vi "CD Init_Prepare Async Data_RT to BC and RT to RT.vi"(8 "error in (no error)":errorcluster, 10 "Card Parameters (in)":T5, 11 "Channels In":T12[](array[typedef]) {"RTs"."Mode Codes"."param item refs" format="%.0x"; "RTs"."Mode Codes"."Timestamp Channel Data Reference" format="%.0x"; "RTs"."subAddresses"."param item refs" format="%.0x"; "RTs"."subAddresses"."Timestamp Channel Data Reference" format="%.0x"; "RTs"."Status Channel Data Reference" format="%.0x"; "RTs"."Command Channels Refs" format="%.0x"; "BC"."Acyclic Frames Trigger Channels Refs" format="%.0x"; "BC"."Command Channels Refs" format="%.0x"; "BC"."messages"."Timestamp Channel Data Reference" format="%.0x"; "BC"."messages"."Status Channel Data Refs" format="%.0x"; "BC"."messages"."param item refs" format="%.0x"; "BC"."messages"."param Block Data Refs"."Data Reference" format="%.0x"}) -> (0 "error out":errorcluster, 1 "param map (RT to BC)":T1, 2 "Raw Values (RT to BC)":T7, 3 "Map (RT to BC)":T9[](array[typedef]) {"Word Data Reference" format="%.0x"})   [LabVIEW 2020, in "Ballard MIL-1553 Engine.lvlib"]
doc: "This VI creates a static association between NI-VS FIFO Channel Index and Physical Channel, Label Index, Parameter Index for Parameter Channel of a Tx Scheduled Label."
uses:
  Ballard MIL-1553 Engine.lvlib
  Shared/Controls and Global/RT Channel.ctl
  Shared/Controls and Global/RT BC.ctl
  <vilib>/NI VeriStand/Custom Device API/Custom Device Item Ref.ctl
  Shared/Controls and Global/RT Message.ctl
  Shared/Controls and Global/RT messageType.ctl
  Shared/Controls and Global/RT CWD1.ctl
  Shared/Controls and Global/RT CWD2.ctl
  <vilib>/NI VeriStand/Custom Device API/Data Reference.ctl
  <vilib>/NI VeriStand/Custom Device API/Block Data Reference.ctl
  System Explorer/SubVIs/Parse Parameters File/param_map_sysdef_type.ctl
  Azdo/emea-ni-vscd_Configurator/source/ConfiguratorConsumer/Ballard_1553/controls/param_type.ctl
  Azdo/emea-ni-vscd_Configurator/source/ConfiguratorConsumer/Ballard_1553/controls/param_signalType_type.ctl
  Azdo/emea-ni-vscd_Configurator/source/ConfiguratorConsumer/Ballard_1553/controls/param_encoding_type.ctl
  Shared/Controls and Global/RT Remote Terminal.ctl
  Shared/Controls and Global/RT Remote Terminal_rtMode.ctl
  Shared/Controls and Global/RT Remote Terminal_RT subAddress.ctl
  Shared/Controls and Global/RT Remote Terminal_RT direction.ctl
  Shared/Controls and Global/RT Remote Terminal_RT Mode Code.ctl
  Controls/RT Async_Map RT2BC.ctl
  Controls/RT Async_Map_Type.ctl
  Controls/RT Async_Raw Values.ctl
  Controls/RT Async_Raw Values to Messages Index_Association.ctl
  Controls/Card Parameters.ctl
  Shared/Controls and Global/Initialization Method.ctl
  Controls/Asynchronous - Parameter map_type.ctl
  Shared/EncodeDecode/_typedefs/parameter_config_type.ctl
  Shared/EncodeDecode/_typedefs/parameter_config_type_type.ctl
  Shared/EncodeDecode/_typedefs/parameter_config_encoding_type.ctl
  Controls/RT Async_Raw Values_Association.ctl
  <instrlib>/BTI1553Lib/Public/Controls/1553 RT Transfer Type.ctl
  <instrlib>/BTI1553Lib/Public/Controls/1553 Transfer Direction.ctl
  <instrlib>/BTI1553Lib/Private/RT/Configure/Get RT Xfer Handle.vi
  <vilib>/NI VeriStand/Custom Device API/Custom Device API.lvlib
  <instrlib>/BTI1553Lib/BTI1553LV.lvlib
  <vilib>/NI VeriStand/Custom Device Tools/Custom Device Utility Library/Custom Device Utility Library.lvlib
  Shared/Ballard 1553 Shared.lvlib
  Azdo/emea-ni-vscd_Configurator/source/ConfiguratorConsumer/Ballard_1553/Ballard_1553.lvclass
  System Explorer/Ballard 1553 System Explorer.lvlib
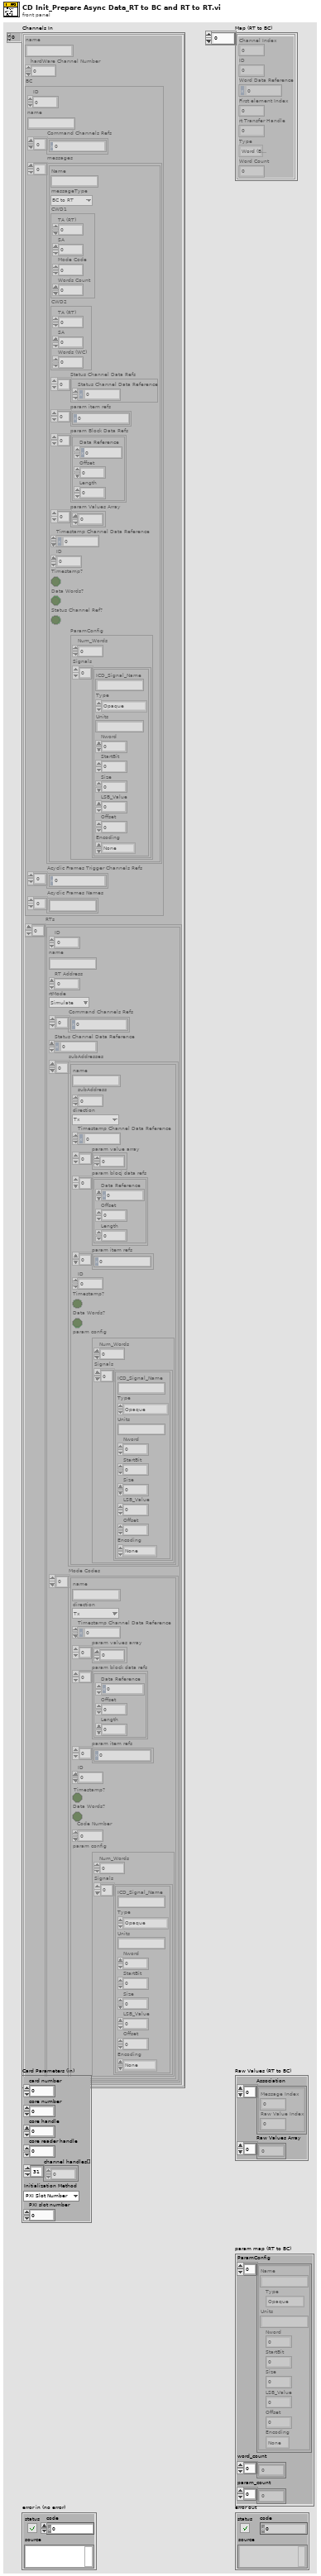
[diagram p1: front panel]
types:
  T1 = typedef "Ballard MIL-1553 Engine.lvlib/Asynchronous - Parameter map_type.ctl" = cluster{"ParamConfig":T2[], "word_count":u8[], "param_count":u8[]}
  T2 = typedef "parameter_config_type.ctl" = cluster{"Name":string, "Type":T3, "Units":string, "Nword":i32, "StartBit":i32, "Size":i32, "LSB_Value":dbl, "Offset":i32, "Encoding":T4}
  T3 = typedef "parameter_config_type_type.ctl" = enum16{"Opaque", "Enum", "Float", "Integer", "Bcd", "Bool"}
  T4 = typedef "parameter_config_encoding_type.ctl" = enum16{"None", "2-complement", "Unsigned"}
  T5 = typedef "Ballard MIL-1553 Engine.lvlib/Card Parameters.ctl" = cluster{"card number":i32, "core number":i32, "core handle":u64, "core reader handle":u64, "channel handles[]":u64[], "Initialization Method":T6, "PXI slot number":i32}
  T6 = typedef "Ballard 1553 Shared.lvlib/Initialization Method.ctl" = enum16{"PXI Slot Number", "Card Number"}
  T7 = typedef "Ballard MIL-1553 Engine.lvlib/RT Async_Raw Values.ctl" = cluster{"Association":T8[], "Raw Values Array":u16[]}
  T8 = typedef "Ballard MIL-1553 Engine.lvlib/RT Async_Raw Values to Messages Index_Association.ctl" = cluster{"Message Index":i32, "Raw Value Index":i32}
  T9 = typedef "Ballard MIL-1553 Engine.lvlib/RT Async_Map RT2BC.ctl" = cluster{"Channel Index":i32, "ID":i32, "Word Data Reference":T10, "First element Index":i32, "rt Transfer Handle":u64, "Type":T11, "Word Count":i32}
  T10 = typedef "Custom Device API.lvlib/Data Reference.ctl" = i32
  T11 = typedef "Ballard MIL-1553 Engine.lvlib/RT Async_Map_Type.ctl" = enum16{"Word (BC to RT)", "Word (MC (Rx))", "Acyclic Message Trigger", "Word (RT to ..)", "Word (RT to RT)", "Word (MC (Tx))", "RT Status", "BC Commands", "RT Commands"}
  T12 = typedef "Ballard 1553 Shared.lvlib/RT Channel.ctl" = cluster{"name":string, "hardWare Channel Number":u16, "BC":T13, "RTs":T24[]}
  T13 = typedef "Ballard 1553 Shared.lvlib/RT BC.ctl" = cluster{"ID":i32, "name":string, "Command Channels Refs":T14[], "messages":T15[], "Acyclic Frames Trigger Channels Refs":T14[], "Acyclic Frames Names":string[]}
  T14 = typedef "Custom Device API.lvlib/Custom Device Item Ref.ctl" = u64
  T15 = typedef "Ballard 1553 Shared.lvlib/RT Message.ctl" = cluster{"Name":string, "messageType":T16, "CWD1":T17, "CWD2":T18, "Status Channel Data Refs":T10[], "param item refs":T14[], "param Block Data Refs":T19[], "param Values Array":u16[], "Timestamp Channel Data Reference":T10, "ID":i32, "Timestamp?":bool, "Data Words?":bool, "Status Channel Ref?":bool, "ParamConfig":T20}
  T16 = typedef "Ballard 1553 Shared.lvlib/RT messageType.ctl" = enum16{"BC to RT", "RT to BC", "RT to RT", "MC (Rx)", "MC (Tx)"}
  T17 = typedef "Ballard 1553 Shared.lvlib/RT CWD1.ctl" = cluster{"TA (RT)":i8, "SA":i8, "Mode Code":i8, "Words Count":i8}
  T18 = typedef "Ballard 1553 Shared.lvlib/RT CWD2.ctl" = cluster{"TA (RT)":i8, "SA":i8, "Words (WC)":i8}
  T19 = typedef "Custom Device API.lvlib/Block Data Reference.ctl" = cluster{"Data Reference":T10, "Offset":u64, "Length":u64}
  T20 = typedef "Ballard 1553 System Explorer.lvlib/param_map_sysdef_type.ctl" = cluster{"Num_Words":u8, "Signals":T21[]}
  T21 = typedef "ConfigurationManager.lvlib/Ballard_1553.lvclass/param_type.ctl" = cluster{"ICD_Signal_Name":string, "Type":T22, "Units":string, "Nword":i32, "StartBit":i32, "Size":i32, "LSB_Value":dbl, "Offset":i32, "Encoding":T23}
  T22 = typedef "ConfigurationManager.lvlib/Ballard_1553.lvclass/param_signalType_type.ctl" = enum16{"Opaque", "Enum", "Float", "Integer", "Bcd", "Bool"}
  T23 = typedef "ConfigurationManager.lvlib/Ballard_1553.lvclass/param_encoding_type.ctl" = enum16{"None", "2-complement", "Unsigned"}
  T24 = typedef "Ballard 1553 Shared.lvlib/RT Remote Terminal.ctl" = cluster{"ID":i32, "name":string, "RT Address":i32, "rtMode":T25, "Command Channels Refs":T14[], "Status Channel Data Reference":T10, "subAddresses":T26[], "Mode Codes":T28[]}
  T25 = typedef "Ballard 1553 Shared.lvlib/RT Remote Terminal_rtMode.ctl" = enum16{"Simulate", "Monitor", "Disable"}
  T26 = typedef "Ballard 1553 Shared.lvlib/RT Remote Terminal_RT subAddress.ctl" = cluster{"name":string, "subAddress":i8, "direction":T27, "Timestamp Channel Data Reference":T10, "param value array":u16[], "param blocj data refs":T19[], "param item refs":T14[], "ID":i32, "Timestamp?":bool, "Data Words?":bool, "param config":T20}
  T27 = typedef "Ballard 1553 Shared.lvlib/RT Remote Terminal_RT direction.ctl" = enum16{"Tx", "Rx"}
  T28 = typedef "Ballard 1553 Shared.lvlib/RT Remote Terminal_RT Mode Code.ctl" = cluster{"name":string, "direction":T27, "Timestamp Channel Data Reference":T10, "param values array":u16[], "param block data refs":T19[], "param item refs":T14[], "ID":i32, "Timestamp?":bool, "Data Words?":bool, "Code Number":i32, "param config":T20}
  T29 = typedef "Ballard MIL-1553 Engine.lvlib/RT Async_Raw Values_Association.ctl" = cluster{"Channel Data Reference":T10, "Raw Value Index":i32}
  T30 = typedef "BTI1553LV.lvlib/1553 Transfer Direction.ctl" = u32
  T31 = typedef "BTI1553LV.lvlib/1553 RT Transfer Type.ctl" = u32
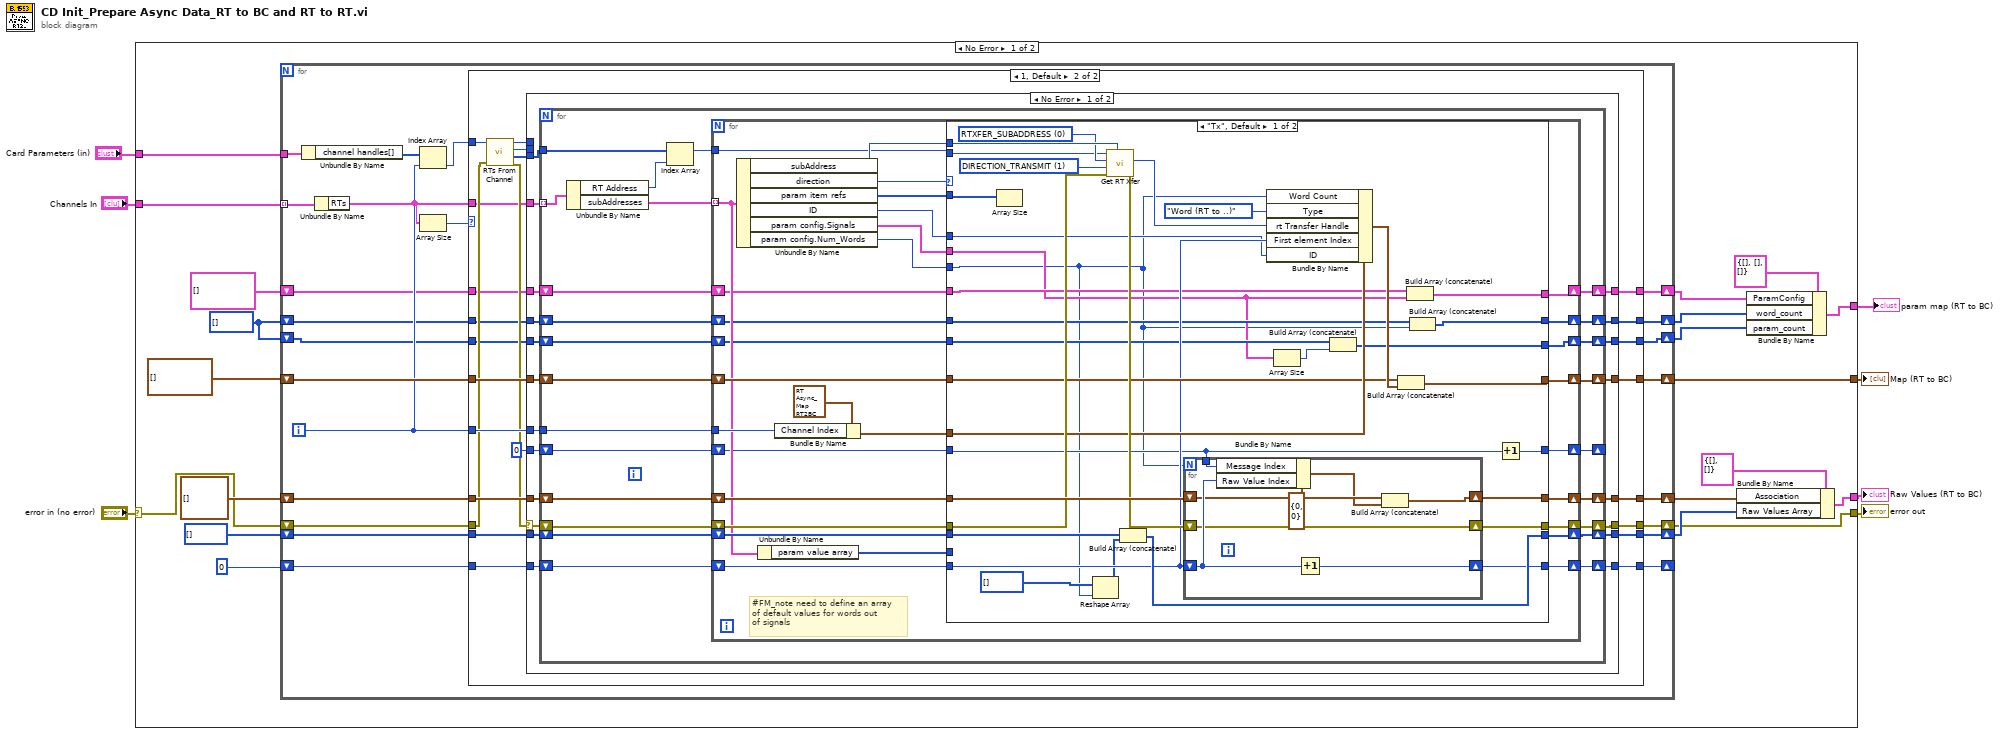
[diagram p0: block diagram]
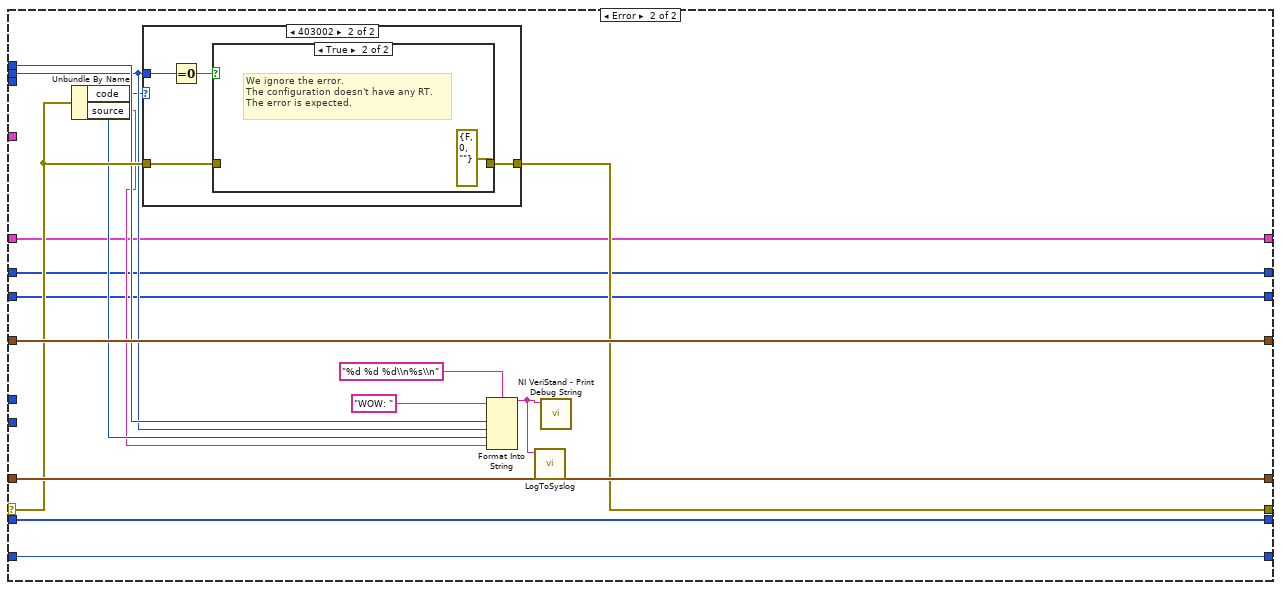
[diagram p4: hidden frame]
diagram:
  n1 = case shown="No Error" "error in (no error)" {
    selector: "error in (no error)" -> [w16 w231]
    tunnel: [w15 w231] -> w6
    tunnel: "Channels In" -> [w27 _]
    tunnel: [w25 _] -> w4
    tunnel: [w21 _] -> w3
    tunnel: "Card Parameters (in)" -> [w17 _]
    tunnel: [w13 _] -> w1
    frame No Error {
      w9 = u8[] [] ("word_count")
      n2 = for {
        tunnel: w27 -> [w50] mode=indexing
        shift-right: [w48] -> w25
        shift-left: T9[] [] -> [w49]
        shift-right: [w46] -> w22
        shift-left: T29[] [] -> [w47]
        shift-right: [w42] -> w19
        shift-left: u16[] [] -> [w45]
        shift-right: [w43] -> _
        shift-left: 0 -> [w44]
        tunnel: w17 -> [w41]
        shift-right: [w38] -> w15
        shift-left: w16 -> [w37]
        shift-right: [w32] -> w11
        shift-left: T2[] [] ("ParamConfig") -> [w33]
        shift-right: [w30] -> w10
        shift-left: w9 -> [w31]
        shift-right: [w28] -> w8
        shift-left: w9 -> [w29]
        i -> [w39]
        n3 = Unbundle By Name(w41) -> ("channel handles[]"=w40:u64[])
        n4 = Unbundle By Name(w50) -> ("RTs"=w35:T24[])
        n5 = Index Array(array=w40, index=w39) -> (element=w36:u64)
        n6 = Array Size(array=w35) -> (size(s)=w34:i32)
        n7 = case shown="1, Default" w34 {
          tunnel: w49 -> [w58 w82]
          tunnel: [w58 w81] -> w48
          tunnel: w47 -> [w57 w80]
          tunnel: [w57 w79] -> w46
          tunnel: w45 -> [w55 w78]
          tunnel: w44 -> [w54 w77]
          tunnel: [w54 w76] -> w43
          tunnel: [w55 w75] -> w42
          tunnel: w39 -> [_ w74]
          tunnel: [w56 w73] -> w38
          tunnel: w37 -> [w56 w72]
          tunnel: w36 -> [_ w67]
          tunnel: w35 -> [_ w66]
          tunnel: w33 -> [w53 w64]
          tunnel: [w53 w63] -> w32
          tunnel: w31 -> [w52 w62]
          tunnel: [w52 w61] -> w30
          tunnel: w29 -> [w51 w60]
          tunnel: [w51 w59] -> w28
          frame 0 {
          }
          frame 1, Default {
            n8 = call <instrlib>:"RTs From Channel.vi"("error in (no error)"=w72, "channel handle in"=w67) -> ("error out"=w69:errorcluster, "remote terminal handles out"=w71:u64[], "remote terminal count out"=w68:i32, "channel handle out"=w65:u64)  [unwired: 6 in]
            n9 = case shown="No Error" w69 {
              selector: w69 -> [w89 w219]
              tunnel: w66 -> [w102 _]
              tunnel: w82 -> [w101 w223]
              tunnel: [w100 w223] -> w81
              tunnel: w80 -> [w99 w222]
              tunnel: [w98 w222] -> w79
              tunnel: w78 -> [w97 w220]
              tunnel: w77 -> [w96 w221]
              tunnel: [w95 w221] -> w76
              tunnel: [w94 w220] -> w75
              tunnel: w74 -> [w93 _]
              tunnel: [w92 w218] -> w73
              tunnel: w71 -> [w91 _]
              tunnel: 0 -> [w90 _]
              tunnel: w68 -> [_ w216]
              tunnel: w65 -> [_ w217]
              tunnel: w64 -> [w88 w210]
              tunnel: [w87 w210] -> w63
              tunnel: w62 -> [w86 w209]
              tunnel: [w85 w209] -> w61
              tunnel: w60 -> [w84 w208]
              tunnel: [w83 w208] -> w59
              frame No Error {
                n10 = for {
                  tunnel: w102 -> [w113] mode=indexing
                  shift-right: [w124] -> w100
                  shift-left: w101 -> [w125]
                  tunnel: w93 -> [w126]
                  shift-right: [w123] -> w98
                  shift-left: w99 -> [w119]
                  shift-right: [w122] -> w94
                  shift-left: w97 -> [w118]
                  shift-right: [w121] -> w95
                  shift-left: w96 -> [w120]
                  tunnel: w91 -> [w117]
                  shift-right: [w115] -> w92
                  shift-left: w89 -> [w116]
                  shift-right: [w109] -> _
                  shift-left: w90 -> [w110]
                  shift-right: [w107] -> w87
                  shift-left: w88 -> [w108]
                  shift-right: [w105] -> w85
                  shift-left: w86 -> [w106]
                  shift-right: [w103] -> w83
                  shift-left: w84 -> [w104]
                  n11 = Unbundle By Name(w113) -> ("RT Address"=w111:i32, "subAddresses"=w114:T26[])
                  n12 = Index Array(array=w117, index=w111) -> (element=w112:u64)
                  n13 = for {
                    tunnel: w126 -> [w156]
                    tunnel: w114 -> [w139] mode=indexing
                    tunnel: w112 -> [w141]
                    shift-right: [w149] -> w121
                    shift-left: w120 -> [w148]
                    shift-right: [w143] -> w115
                    shift-left: w116 -> [w144]
                    shift-right: [w154] -> w124
                    shift-left: w125 -> [w155]
                    shift-right: [w151] -> w123
                    shift-left: w119 -> [w147]
                    shift-right: [w150] -> w122
                    shift-left: w118 -> [w146]
                    shift-right: [w136] -> w109
                    shift-left: w110 -> [w137]
                    shift-right: [w134] -> w107
                    shift-left: w108 -> [w135]
                    shift-right: [w132] -> w105
                    shift-left: w106 -> [w133]
                    shift-right: [w130] -> w103
                    shift-left: w104 -> [w131]
                    # "#FM_note need to define an array\nof default values for words out \nof signals"
                    n14 = Unbundle By Name(w139) -> ("subAddress"=w142:i8, "direction"=w138:T27, "param item refs"=w152:T14[], "ID"=w129:i32, "param config.Signals"=w127:T21[], "param config.Num_Words"=w128:u8)
                    n15 = Unbundle By Name(w139) -> ("param value array"=w145:u16[])
                    n16 = Bundle By Name(cluster=T9 {"Channel Index"=0, "ID"=0, "Word Data Reference"=0, "First element Index"=0, "rt Transfer Handle"=0, "Type"=enum."Word (BC to RT)", "Word Count"=0} ("Association"), "Channel Index"=w156) -> (w153:T9)
                    n17 = case shown="\"Tx\", Default" w138 {
                      tunnel: w155 -> [w174 w207]
                      tunnel: [w173 w207] -> w154
                      tunnel: w153 -> [w178 _]
                      tunnel: w152 -> [w171 _]
                      tunnel: [w179 w206] -> w151
                      tunnel: [w190 w204] -> w150
                      tunnel: [w189 w203] -> w149
                      tunnel: w148 -> [w170 w203]
                      tunnel: w147 -> [w188 w206]
                      tunnel: w146 -> [w187 w204]
                      tunnel: w145 -> [_ _]
                      tunnel: w144 -> [w186 w205]
                      tunnel: [w184 w205] -> w143
                      tunnel: w142 -> [w183 _]
                      tunnel: w141 -> [w181 _]
                      tunnel: w137 -> [w169 w202]
                      tunnel: [w172 w202] -> w136
                      tunnel: w135 -> [w168 w201]
                      tunnel: [w167 w201] -> w134
                      tunnel: w133 -> [w166 w200]
                      tunnel: [w165 w200] -> w132
                      tunnel: w131 -> [w161 w199]
                      tunnel: [w160 w199] -> w130
                      tunnel: w129 -> [w159 _]
                      tunnel: w128 -> [w157 _]
                      tunnel: w127 -> [w158 _]
                      frame "Tx", Default {
                        w180 = T30 1 items=["DIRECTION_RECEIVE", "DIRECTION_TRANSMIT"] ("transfer direction")
                        w182 = T31 0 items=["RTXFER_SUBADDRESS", "RTXFER_MODECODE"] ("transfer type")
                        n18 = Array Size(array=w171) -> ()  [unwired: 1 out]
                        n19 = Reshape Array(u16[] [] ("param value array"), w157) -> (w163:u16[])
                        n20 = call-poly <instrlib>:"Get RT Xfer.vi"("transfer sa number or mc number"=w183, "error in (no error)"=w186, "transfer direction"=w180, "transfer type"=w182, "remote terminal handle in"=w181) -> ("error out"=w185:errorcluster, "rt transfer handle out"=w176:u64)  [unwired: 4 in, 1 out]
                        n21 = Build Array (concatenate)(w187, w163) -> (w190:u16[])
                        n22 = for {
                          N: w157 -> [_]
                          shift-right: [w198] -> w189
                          shift-left: w170 -> [w197]
                          shift-right: [w195] -> w184
                          shift-left: w185 -> [w195]
                          shift-right: [w192] -> w179
                          shift-left: w188 -> [w196]
                          tunnel: w169 -> [w191]
                          n23 = Bundle By Name(cluster=T8 {"Message Index"=0, "Raw Value Index"=0}, "Message Index"=w191, "Raw Value Index"=w197) -> (w193:T8)
                          n24 = Increment(x=w197) -> (x+1=w198:i32)
                          n25 = Build Array (concatenate)(w196, w193) -> (w192:T29[])
                        }
                        n26 = Bundle By Name(cluster=w178, "Word Count"=w157, "Type"=RT_Async_Map_Type."Word (RT to ..)", "rt Transfer Handle"=w176, "First element Index"=w170, "ID"=w159) -> (w175:T9)
                        n27 = Array Size(array=w158) -> (size(s)=w162:i32)
                        n28 = Build Array (concatenate)(w161, w162) -> (w160:i32[])
                        n29 = Build Array (concatenate)(w174, w175) -> (w173:T9[])
                        n30 = Build Array (concatenate)(w168, w158) -> (w167:T21[])
                        n31 = Build Array (concatenate)(w166, w157) -> (w165:u8[])
                        n32 = Increment(x=w169) -> (x+1=w172:i32)
                      }
                      frame "Rx" {
                      }
                    }
                  }
                }
              }
              frame Error {
                n33 = Unbundle By Name(w219) -> ("code"=w215:i32, "source"=w214:string)
                n34 = case shown="403002" w215 {
                  tunnel: w219 -> [w224 w226]
                  tunnel: w216 -> [_ w228]
                  tunnel: [w224 w225] -> w218
                  frame 0, Default {
                  }
                  frame 403002 {
                    n35 = Equal To 0?(x=w228) -> (x = 0?=w227:bool)
                    n36 = case shown="True" w227 {
                      tunnel: w226 -> [w229 _]
                      tunnel: [w229 errorcluster {"status"=FALSE, "code"=0, "source"=""} ("error IO")] -> w225
                      frame False {
                      }
                      frame True {
                        # "We ignore the error.\nThe configuration doesn't have any RT.\nThe error is expected."
                      }
                    }
                  }
                }
                n37 = Format Into String(format string="%d %d %d\\n%s\\n", initial string="WOW: ", w217, w216, w215, w214) -> (resulting string=w211:string)  [unwired: 1 in, 1 out]
                n38 = call "LogToSyslog.vi"("message"=w211) -> ()  [unwired: 9 in, 2 out]
                n39 = call <vilib>:"NI VeriStand - Print Debug String.vi"("Message"=w211) -> ()  [unwired: 10 in, 1 out]
              }
            }
          }
        }
      }
      n40 = Bundle By Name(cluster=T7 {"Association"=[], "Raw Values Array"=[]} ("Raw Values"), "Association"=w22, "Raw Values Array"=w19) -> (w21:T7)
      n41 = Bundle By Name(cluster=T1 {"ParamConfig"=[], "word_count"=[], "param_count"=[]}, "ParamConfig"=w11, "word_count"=w10, "param_count"=w8) -> (w13:T1)
    }
    frame Error {
    }
  }
  "error out" <- w6
  "Map (RT to BC)" <- w4
  "Raw Values (RT to BC)" <- w3
  "param map (RT to BC)" <- w1
